vi "Tecella_CmdLine.vi"() -> ()   [LabVIEW 2009]
uses:
  TecellaClient/TecellaClient.lvclass
panel:
  in  "stop":bool
  out "Data Returned":string
  in  "data in":string="GET /help/map.htm HTTP/1.1\nHost: www.ni.com\n\n"
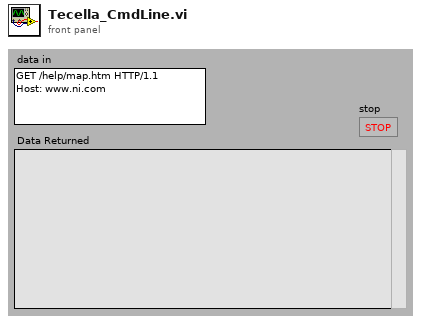
[diagram p1: front panel]
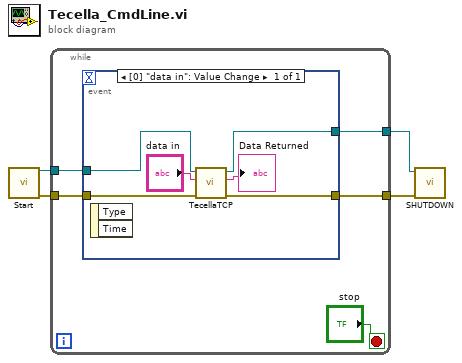
[diagram p0: block diagram]
diagram:
  n1 = call "Start.vi"() -> ("TecellaClient"=w4:refnum<class "TecellaClient.lvclass">, "error out"=w3:errorcluster)  [unwired: 11 in, 3 out]
  n2 = while {
    tunnel: w4 -> [w9]
    tunnel: w3 -> [w8]
    tunnel: [w7] -> w2
    tunnel: [w6] -> w1
    stop <- "stop" stop-if-true
    n3 = event shown="[0] \"data in\": Value Change" {
      selector: _ -> [_]
      dyn-events: _ -> [_]
      timeout: _ -> [_]
      tunnel: w9 -> [w15]
      tunnel: w8 -> [w14]
      tunnel: [w13] -> w7
      tunnel: [w12] -> w6
      event [0] "data in": Value Change {
        n4 = event-data() -> ()  [unwired: 1 in, 2 out]
        n5 = call-dynamic "TecellaTCP.vi"("error in (no error)"=w14, "data in"="data in", "TecellaClient in"=w15) -> ("error out"=w12:errorcluster, "Data Returned"=→"Data Returned":string, "TecellaClient out"=w13:refnum<class "TecellaClient.lvclass">)  [unwired: 6 in]
      }
    }
  }
  n6 = call-dynamic "SHUTDOWN.vi"("error in (no error)"=w1, "TecellaClient in"=w2) -> ()  [unwired: 8 in, 2 out]
